vi "Software PWM Real.vi"(9 "Duty Cycle (0-100)":dbl, 10 "Steps":dbl, 11 "Cycle Time (s)":dbl) -> (3 "Waveform Chart 2":i16(graph))   [LabVIEW 2011]
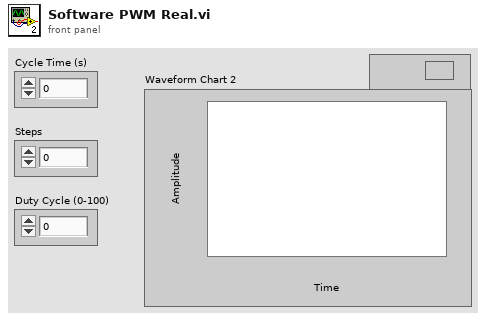
[diagram p1: front panel]
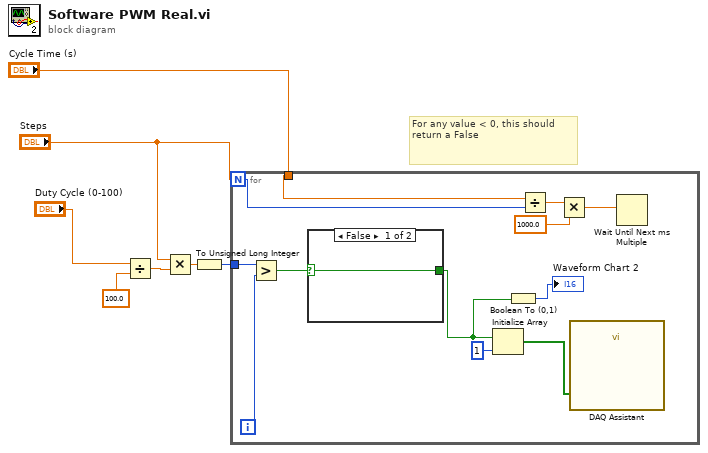
[diagram p0: block diagram]
diagram:
  # "For any value < 0, this should return a False"
  n1 = Divide(x="Duty Cycle (0-100)", y=100.0) -> (x/y=w4:dbl)
  n2 = Multiply(x="Steps", y=w4) -> (x*y=w6:dbl)
  n3 = To Unsigned Long Integer(number=w6) -> (unsigned 32bit integer=w7:u32)
  n4 = for {
    N: "Steps" -> [w16]
    tunnel: "Cycle Time (s)" -> [w15]
    tunnel: w7 -> [w14]
    i -> [w13]
    n5 = Greater?(x=w14, y=w13) -> (0:w12:bool)
    n6 = case shown="False" w12 {
      selector: w12 -> [w20 w21]
      tunnel: [w20 w21] -> w9
      frame False {
      }
      frame True {
      }
    }
    n7 = Initialize Array(w9, 1 ("dimension size")) -> (w10:bool[])
    n8 = Boolean To (0,1)(Boolean=w9) -> (0, 1=→"Waveform Chart 2":i16)
    n9 = Divide(x=w15, y=w16) -> (x/y=w19:dbl)
    n10 = Multiply(x=w19, y=1000.0) -> (x*y=w17:dbl)
    n11 = call "DAQ Assistant"("data"=w10) -> ()  [unwired: 17 in, 2 out]
    n12 = Wait Until Next ms Multiple(millisecond multiple=w17) -> ()  [unwired: 1 out]
  }
